vi "Check Aircraft Telem Port.vi"(8 "Error In":errorcluster, 11 "Aircraft ID":u8) -> (0 "Error Out":errorcluster, 3 "Telem Port Found":bool)   [LabVIEW 2014]
uses:
  Get Aircraft Information.vi
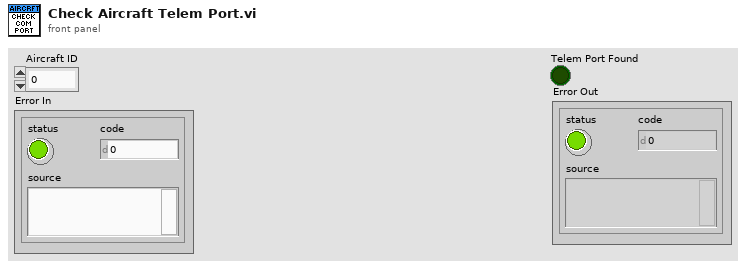
[diagram p1: front panel]
types:
  T1 = typedef "Drone Information.ctl" = cluster{"Heart Beat":bool, "Aircraft ID":u8, "Downlink Port":refnum<visa-resource-name>, "Tag ID":string, "System Status":string, "Base Mode":T2, "Armed/Disarmed":bool, "Battery Voltage":dbl, "Control Mode":T3, "Initialisation":u8, "Heart Beat Status":bool, "Uplink Port":refnum<visa-resource-name>, "UDP connection ID":refnum<k16>, "Connection Type":T4, "Mode":string, "UDP IP Address":string, "Mission Uploaded":bool}
  T2 = typedef "Base Mode.ctl" = cluster{"Custom Mode":bool, "Test Enabled":bool, "Autonomous Mode":bool, "Guided Mode":bool, "Stabilization Enabled":bool, "HIL Enabled":bool, "Manual Mode":bool, "Arm":bool}
  T3 = typedef "Aircraft Mode.ctl" = enum16{"Loiter", "Stabalise", "Failsafe", "Emergency Stop"}
  T4 = typedef "Telemetry Connection Type.ctl" = enum16{"Serial", "UDP", "TCP"}
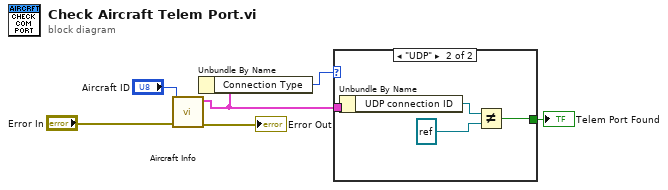
[diagram p0: block diagram]
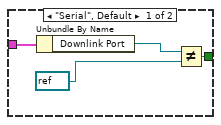
[diagram p2: hidden frame]
diagram:
  n1 = call-poly "Aircraft Info.vi"("Error In"="Error In", "Aircraft ID"="Aircraft ID") -> ("Error Out"=→"Error Out":errorcluster, "Aircraft Information Out"=w2:T1)  [unwired: 8 in]
  n2 = Unbundle By Name(w2) -> ("Connection Type"=w1:T4)
  n3 = case shown="\"UDP\"" w1 {
    tunnel: w2 -> [w10 w14]
    tunnel: [w7 w12] -> w5
    frame "Serial", Default {
      n4 = Unbundle By Name(w10) -> ("Downlink Port"=w9:refnum<visa-resource-name>)
      n5 = Not Equal?(x=w9, y=refnum<visa-resource-name> refnum ("Communication Port")) -> (x != y?=w7:bool)
    }
    frame "UDP" {
      n6 = Unbundle By Name(w14) -> ("UDP connection ID"=w13:refnum<k16>)
      n7 = Not Equal?(x=w13, y=refnum<k16> refnum) -> (x != y?=w12:bool)
    }
  }
  "Telem Port Found" <- w5
